vi "Dashboard Main.vi"() -> ()   [LabVIEW 2013]
uses:
  subStates.ctl
  <vilib>/event_ctls.llb/eventvkey.ctl
  dash dio.ctl
  misc dash data.ctl
  dashboard safety status data.ctl
  dash error type def.ctl
  <vilib>/Utility/config.llb/Write Key (String).vi
  <vilib>/Utility/config.llb/Write Key (I32).vi
  <vilib>/Utility/config.llb/NI_LVConfig.lvlib
panel:
  out "Image Message":string="Timeout in Camera Communications"
  in  "Dashboard Tab":T1(tab)
  out "no rate":bool
  out "arm encoder limit":bool
  out "hold":bool
  out "shoot?":bool
  out "Shifter":bool
  out "Vision State":bool
  in  "Camera Settings":T2={"Frame Rate"=30, "Compression"=30, "Size"=1} {"Frame Rate" scale=1.0..30.0; "Size" items=["640x480", "320x240", "160x120"]}
  out "Mode":T3(ring)=enum."Auto Disabled"
  out "Camera IP":string
  in  "DB Camera Config":bool
  out "fps":dbl format="%#.1g"
  out "Mbps":dbl format="%#.1g"
  out "Mbps 2":bool
  out "Distance From Target":dbl
  out "Hot Goal Present?":bool
  out "arm saftey":bool
  out "Directional Failure":bool
  out "timeout error":bool
  out "# of Timeouts":u32
  out "Robot IP\nAddress":string
  out "Solenoid Output":bool[](array[boolean])
  out "PWM":cluster{u8, u8}[](array[slide])=[{0, 157}, {0, 157}, {0, 157}, {0, 157}, {0, 157}, {0, 157}, {0, 157}, {0, 157}, {0, 157}, {0, 169}] scale=1.0..255.0
  out "GPIO Output Enable":bool[](array[boolean])
  out "GPIO State":bool[](array[boolean])
  out "Relay":cluster{"Forward":bool[], "Reverse":bool[]}
  out "8 -- Battery":sgl(graph)
  out "Analog Input":sgl[](array[slide]) scale=0.0..5.0
  out "Drive":T4
  out "Pickup/Passing \nArm":cluster{"Distance ":dbl, "Rate":dbl}
  out "Latch":T5
  out "Pickup Arm":T5
  out "Belts":T5
  out "Shooter":T5
  out "Drive":T5
  out "Belt Status":u16(ring) items=["Code Control", "Driver Control", "Manual Override"]
  out "Arm Status":u16(ring) items=["Code Control", "Driver Control", "Manual Override"]
  out "Belts":dbl
  out "CPU":dbl(slide) scale=0.0..100.0
  out "cRIO CPU Usage":dbl(knob) scale=0.0..100.0
  out "Code Iterations Per Second":cluster{dbl, dbl}(knob) scale=0.0..60.0
  out "Vision mSPI":u32
  out "Main mSPI":u32
  in  "Listbox":i32(listbox)
  out "Tree":string(tree)
  in  "Enable":bool
  # "ft"
  # "Encoders"
  # "States"
  # "Drive"
  # "Belts"
  # "Communications"
  # "Solenoid #1"
  # "1"
  # "8"
  # "Digital #1"
  # "1"
  # "10"
  # "1"
  # "14"
  # "1"
  # "8"
  # "Analog #1"
  # "1"
  # "7"
  # "Main IPS"
  # "Vision IPS"
  # "Grey - Vision\nBlack - Main"
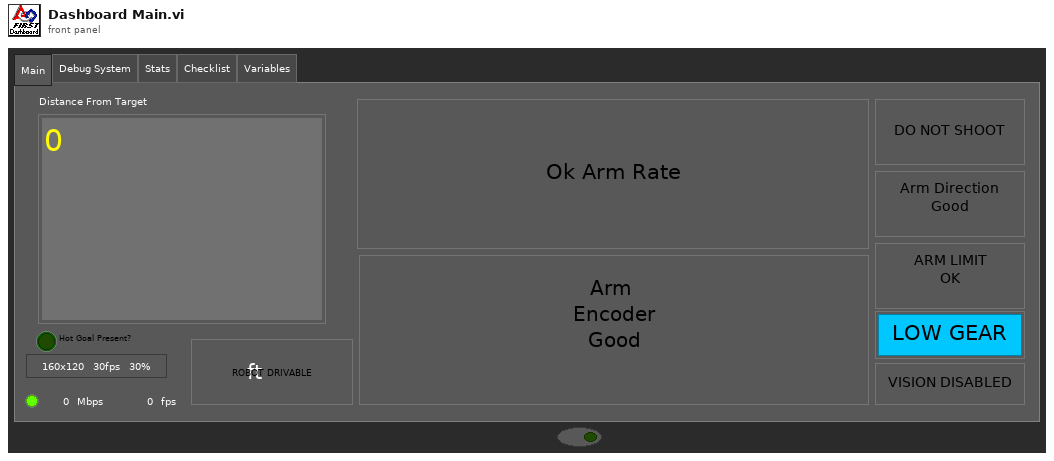
[diagram p1: front panel]
types:
  T1 = enum32{"Main", "Debug System", "Stats", "Checklist", "Variables"}
  T2 = cluster{"Frame Rate":i32, "Compression":i32, "Size":u16}
  T3 = enum8{"Tele-Op Disabled", "Tele-Op Enabled", "Auto Disabled", "Auto Enabled", "Test Disabled", "Test Enabled", ""}
  T4 = cluster{"Right Rate":dbl, "Left Rate":dbl, "Left Distance":dbl, "Right Distance":dbl}
  T5 = typedef "subStates.ctl" = enum16{"null", "wait", "driver control", "auto", "manual override", "hold position", "rotate", "pickup", "pass", "load", "goto shoot", "shoot", "end", "test"}
  T6 = typedef "Image Type" = u32
  T7 = typedef "IMAQ Image.ctl" = refnum<image>
  T8 = typedef "dash error type def.ctl" = cluster{"Timeout Data":cluster{"# of Timeouts":u32, "Time Out Error This Match":bool}, "Can Shoot Safely?":bool}
  T9 = typedef "misc dash data.ctl" = cluster{"Total (%)":dbl, "Vision mSPI":u32, "Main mSPI":u32, "Vision":cluster{"Hot Goal Present?":bool, "distance":dbl}, "Enabled?":bool, "Safety Data":T10}
  T10 = typedef "dashboard safety status data.ctl" = cluster{"At Distance Limit":bool, "Encoder Error":bool, "Excedded Rate Limit":bool, "Encoder Directional Issue":bool}
  T11 = typedef "dash dio.ctl" = cluster{"Relay Forward":u8, "Relay Reverse":u8, u32, u32, cluster{"[0]":u8, "[1]":u8, "[2]":u8, "[3]":u8, "[4]":u8, "[5]":u8, "[6]":u8, "[7]":u8, "[8]":u8, "[9]":u8}}[]
  T12 = cluster{"Digital Inputs":bool[], "Digital Outputs":bool[]}
  T13 = cluster{"Competition mode":bool, "Robot Link":bool, "Autonomous":bool, "Enabled":bool, "E-Stop":bool, "Simulated":bool, "TestMode":bool, "Docked Window":bool}
  T14 = cluster{"Relay Forward":u8, "Relay Reverse":u8, u32, u32, cluster{"[0]":u8, "[1]":u8, "[2]":u8, "[3]":u8, "[4]":u8, "[5]":u8, "[6]":u8, "[7]":u8, "[8]":u8, "[9]":u8}}
  T15 = cluster{"Hot Goal Present?":bool, "distance":dbl}
  T16 = cluster{"# of Timeouts":u32, "Time Out Error This Match":bool}
  T17 = cluster{"Numeric":dbl, "Numeric":dbl, "Numeric":dbl, "Numeric":dbl}
  T18 = typedef "NI_LVConfig.lvlib/Config Data RefNum.ctl" = refnum<k1>
  T19 = typedef "eventvkey.ctl" = enum16{"ASCII", "Enter", "Return", "Shift", "Ctrl", "Alt", "Cmd", "Opt", "Caps", "NumLock", "Clear", "Break", "Up", "Down", "Left", "Right", "Insert", "Delete", "Home", "End", "PageUp", "PageDown", "Escape", "Help", "Pause", "ScrollLock", "F1", "F2", "F3", "F4", "F5", "F6", "F7", "F8", "F9", "F10", "F11", "F12", "F13", "F14", "F15", "F16", "F17", "F18", "F19", "F20", "F21", "F22", "F23", "F24", "Play", "VolumeUp", "VolumeDown", "Mute", "Two Byte Char"}
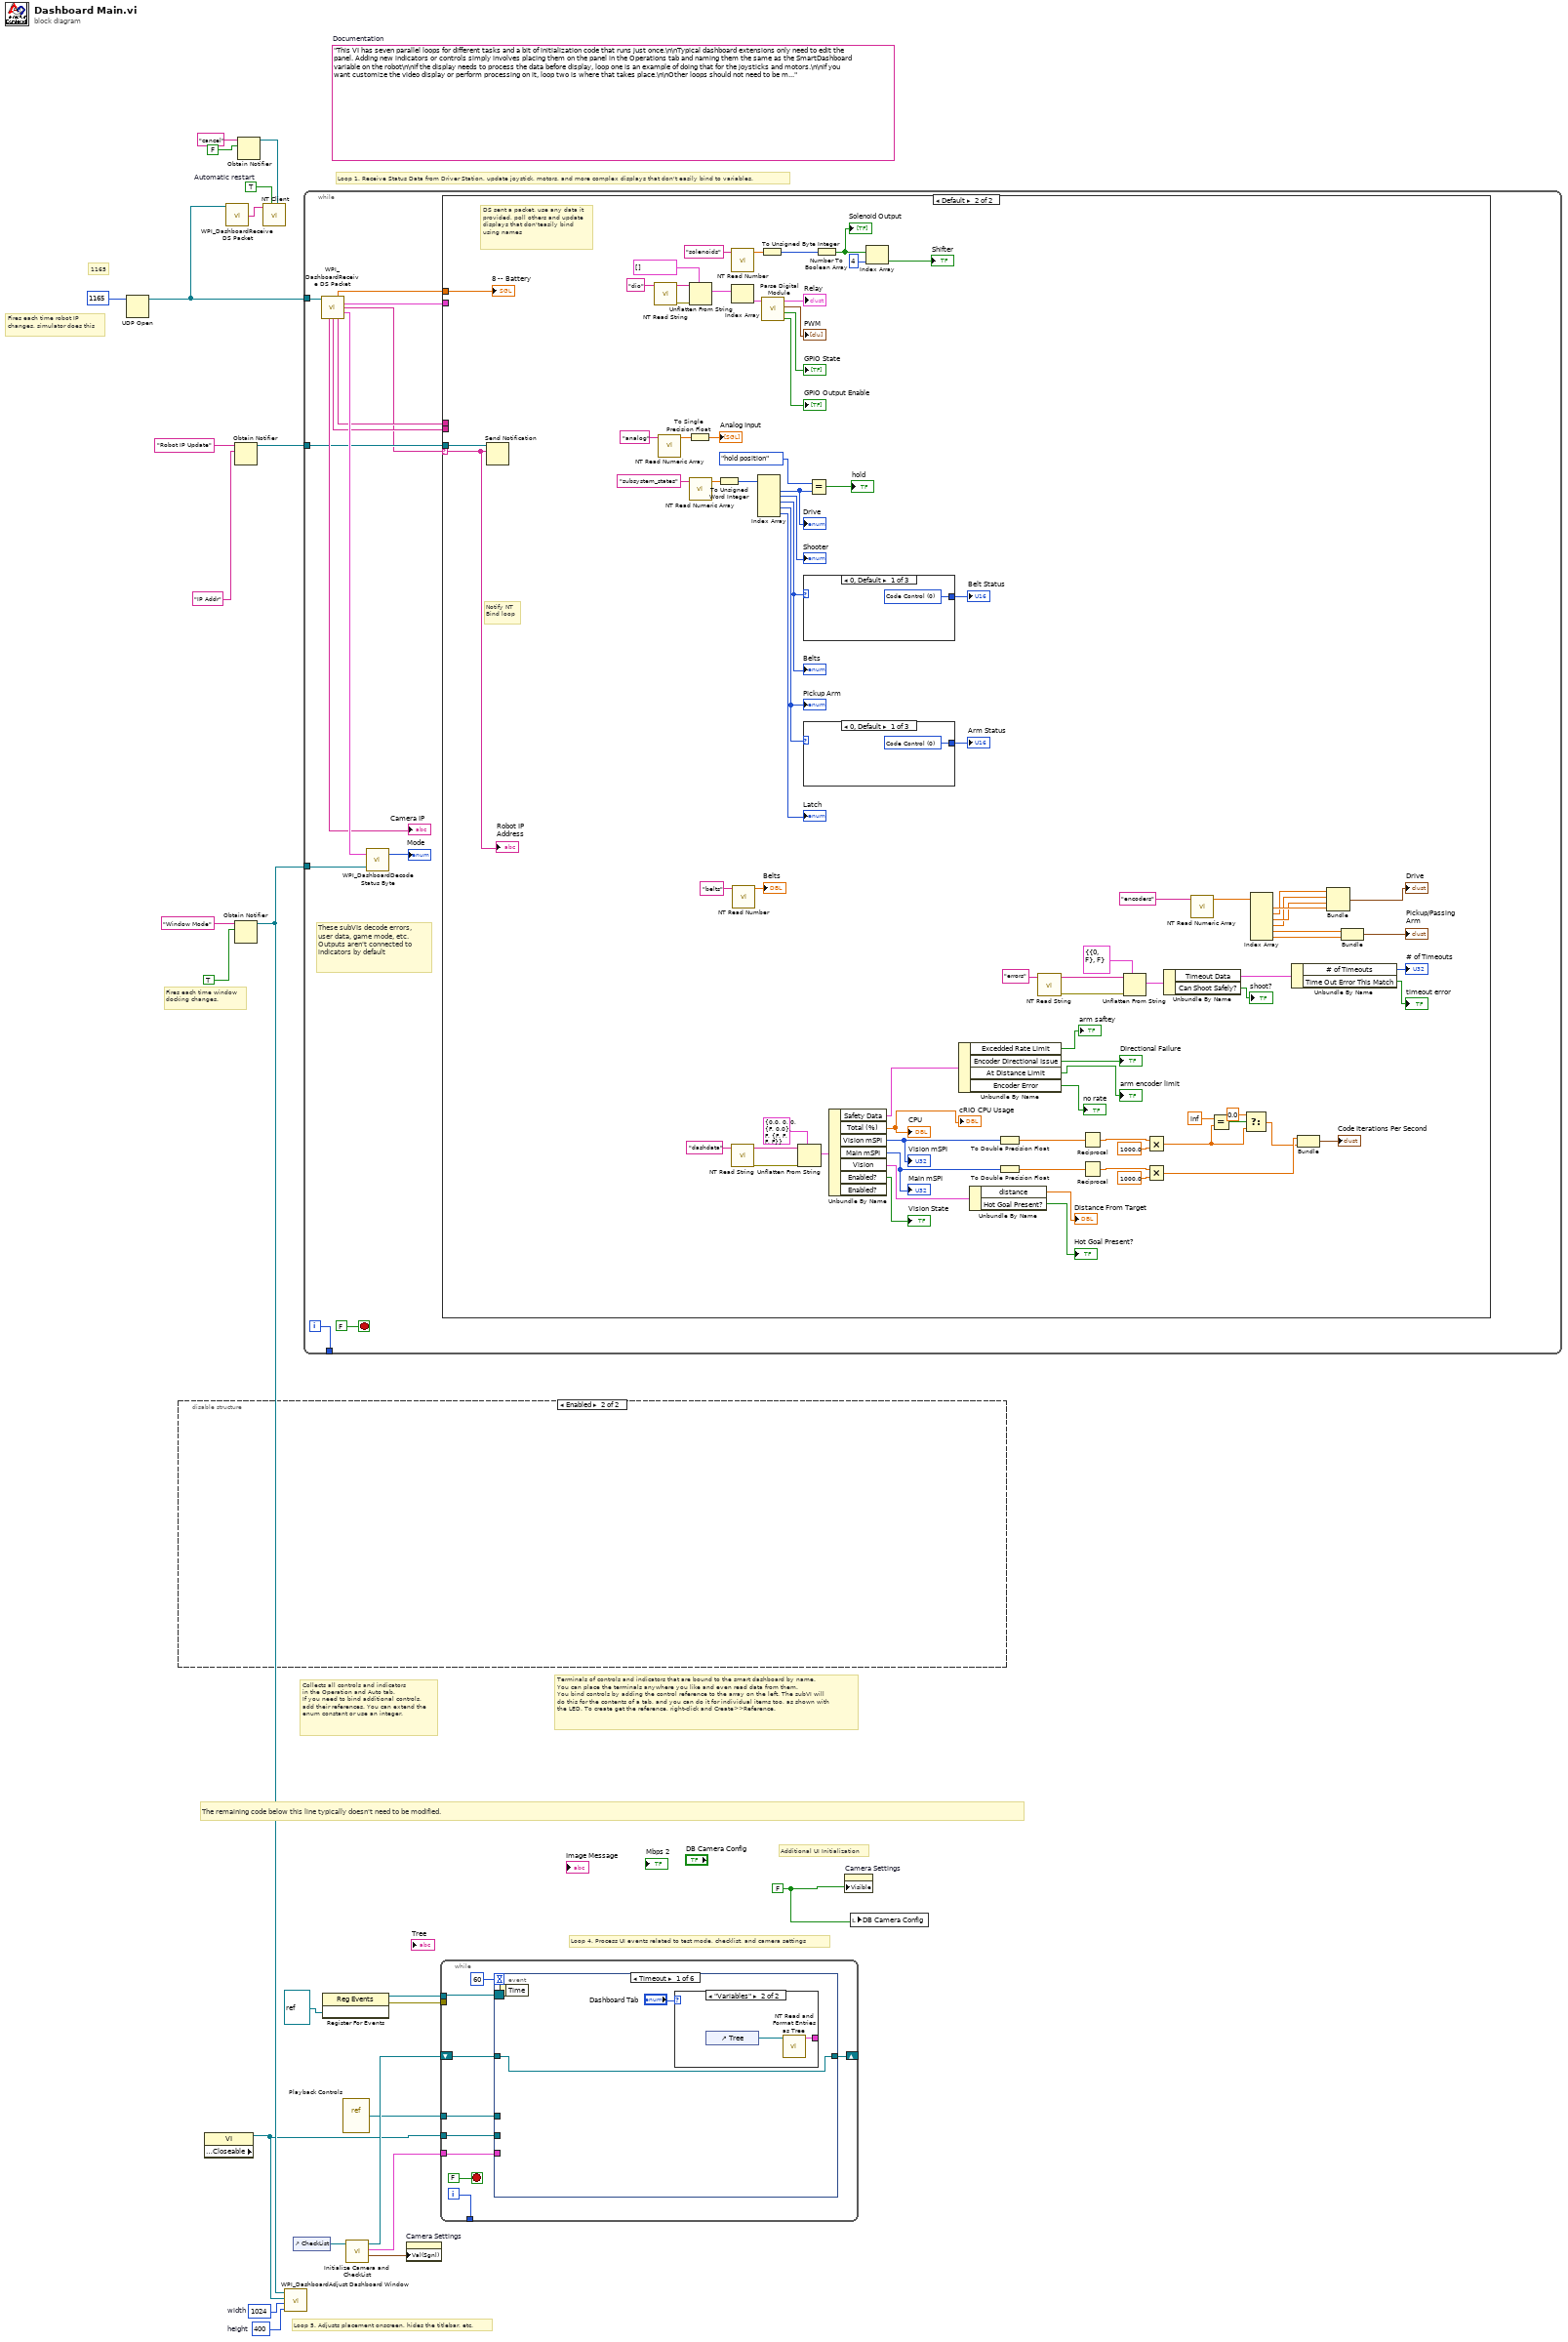
[diagram p0: block diagram]
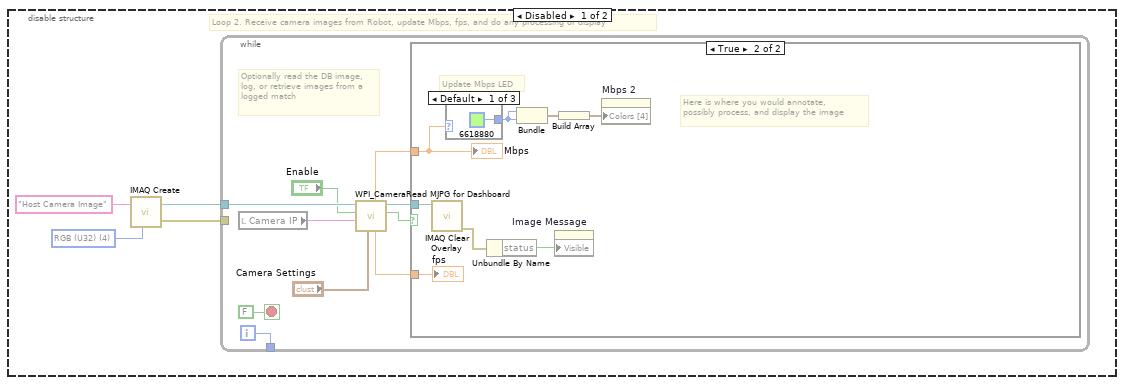
[diagram p2: hidden frame]
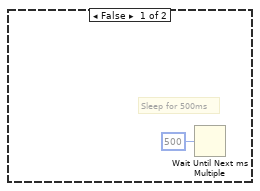
[diagram p3: hidden frame]
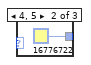
[diagram p4: hidden frame]
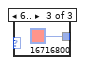
[diagram p5: hidden frame]
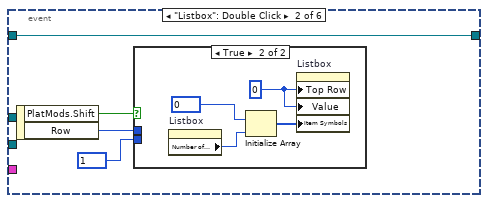
[diagram p7: hidden frame]
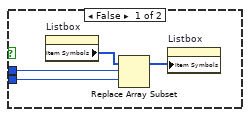
[diagram p8: hidden frame]
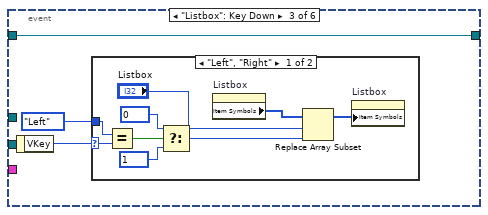
[diagram p9: hidden frame]
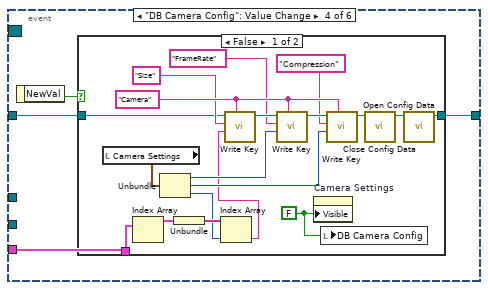
[diagram p11: hidden frame]
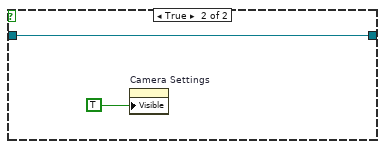
[diagram p12: hidden frame]
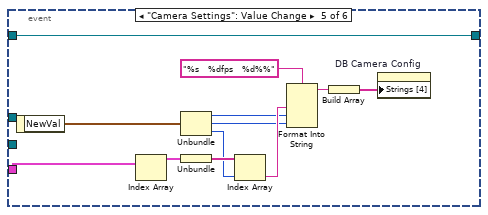
[diagram p13: hidden frame]
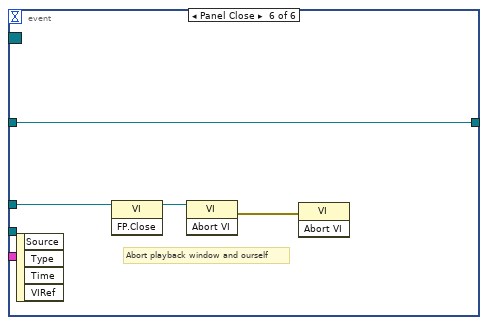
[diagram p14: hidden frame]
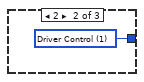
[diagram p16: hidden frame]
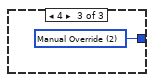
[diagram p17: hidden frame]
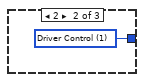
[diagram p18: hidden frame]
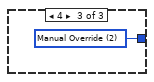
[diagram p19: hidden frame]
diagram:
  w6 = TRUE  # Automatic restart
  w9 = 400  # height
  w10 = 1024  # width
  w19 = FALSE ("Visible")
  (unwired) "This VI has seven parallel loops for different tasks and a bit of initialization code that runs just once.\n\nTypical dashboard extensions only need to edit the panel. Adding new indicators or controls simply involves placing them on the panel in the Operations tab and naming them the same as the SmartDashboard variable on the robot\n\nIf the display needs to process the data before display, loop one is an example of doing that for the joysticks and motors.\n\nIf you want customize the video display or perform processing on it, loop two is where that takes place.\n\nOther loops should not need to be modified. They are pretty standard, and document the task they perform."  # Documentation
  # "1165"
  # "Loop 4. Process UI events related to test mode, checklist, and camera settings"
  # "Loop 5. Adjusts placement onscreen, hides the titlebar, etc."
  # "Additional UI Initialization"
  # "Fires each time robot IP\nchanges, simulator does this"
  # "Fires each time window\ndocking changes."
  # "Collects all controls and indicators\nin the Operation and Auto tab.\nIf you need to bind additional controls,\nadd their references. You can extend the\nenum constant or use an integer."
  # "The remaining code below this line typically doesn't need to be modified."
  # "Terminals of controls and indicators that are bound to the smart dashboard by name.\nYou can place the terminals anywhere you like and even read data from them.\nYou bind controls by adding the control reference to the array on the left. The subVI will\ndo this for the contents of a tab, and you can do it for individual items too, as shown with\nthe LED. To create get the reference, right-click and Create>>Reference."
  # "Loop 1. Receive Status Data from Driver Station, update joystick, motors, and more complex displays that don't easily bind to variables."
  n1 = UDP Open(11:u16 1165 ("port")) -> (port=w1:refnum<k16>)  [unwired: 2 in, 4 out]
  n2 = disable-structure shown="Enabled" {
    frame Disabled {
      w29 = T6 4 items=["Grayscale (U8)", "Grayscale (I16)", "Grayscale (SGL)", "Complex (CSG)", "RGB (U32)", "HSL (U32)", "RGB (U64)"] ("Image Type")
      # "Loop 2. Receive camera images from Robot, update Mbps, fps, and do any processing or display"
      n3 = call "IMAQ Create"("Image Name"="Host Camera Image", "Image Type"=w29) -> ("New Image"=w27:T7, "error out"=w26:errorcluster)  [unwired: 2 in, 1 out]
      n4 = while {
        tunnel: w27 -> [w37]
        tunnel: w26 -> [_]
        tunnel: [w38] -> _
        i -> [w38]
        stop <- FALSE stop-if-true
        # "Optionally read the DB image,\nlog, or retrieve images from a\nlogged match"
        n5 = local read "Camera IP"() -> (w30:string)
        n6 = call <vilib>:"WPI_CameraRead MJPG for Dashboard.vi"("Camera Settings"="Camera Settings", "Camera IP"=w30, "Enable"="Enable", "Refnum in"=w37) -> ("Active"=w34:bool, "Refnum out"=w36:T7, "FPS"=w33:dbl, "Bandwidth (Mbps)"=w32:dbl)  [unwired: 4 in]
        n7 = case shown="True" w34 {
          tunnel: w36 -> [_ w44]
          tunnel: w32 -> [_ w43]
          tunnel: w33 -> [_ w41]
          frame False {
            # "Sleep for 500ms"
            n8 = Wait Until Next ms Multiple(millisecond multiple=u32 500) -> ()  [unwired: 1 out]
          }
          frame True {
            # "Here is where you would annotate,\npossibly process, and display the image"
            # "Update Mbps LED"
            n9 = call "IMAQ Clear Overlay"("Image"=w44) -> ("error out"=w48:errorcluster, "Image Out"=w42:T7)  [unwired: 2 in, 7 out]
            n10 = case shown="Default" w43 {
              tunnel: [u32 6618880 ("Color Box") u32 16776722 ("Color Box") u32 16716800 ("Color Box")] -> w45
              frame Default {
              }
              frame 4, 5 {
              }
              frame 6.. {
              }
            }
            n11 = Unbundle By Name(w48) -> ("status"=w49:bool)
            n12 = Bundle("Color Box"=w45, "Color Box"=w45) -> (w47:cluster{"Color Box":u32, "Color Box":u32})  [unwired: 1 out]
            n13 = property on="Image Message" class="Str"("Visible"=w49) -> ()  [unwired: 2 in, 2 out]
            n14 = Build Array(w47) -> (w46:cluster{"Color Box":u32, "Color Box":u32}[])
            n15 = property on="Mbps 2" class="Bool (strict)"("Colors [4]"=w46) -> ()  [unwired: 2 in, 2 out]
            "Mbps" <- w43
            "fps" <- w41
          }
        }
      }
    }
    frame Enabled {
    }
  }
  n16 = property class="VI" props=["Front Panel.Closeable"]() -> (reference out=w7:refnum<vi>)  [unwired: 2 in, 2 out]
  n17 = call <vilib>:"WPI_DashboardReceive DS Packet.vi"("Recv Socket"=w1) -> ("Robot IP Address"=w2:string)  [unwired: 1 in, 13 out]
  n18 = Obtain Notifier(name (unnamed)="Robot IP Update", notification data type="IP Addr" ("name (unnamed)")) -> (notifier out=w22:refnum<notifier>)  [unwired: 2 in, 2 out]
  n19 = Obtain Notifier(name (unnamed)="Window Mode", notification data type=TRUE) -> (notifier out=w18:refnum<notifier>)  [unwired: 2 in, 2 out]
  n20 = Obtain Notifier(name (unnamed)="cancel", notification data type=FALSE) -> (notifier out=w3:refnum<notifier>)  [unwired: 2 in, 2 out]
  n21 = call <vilib>:"NT Client.vi"("Cancel Ref"=w3, "Automatic restart"=w6, "Server IP Address"=w2) -> ()  [unwired: 9 in]
  n22 = call <vilib>:"WPI_DashboardAdjust Dashboard Window.vi"("height"=w9, "width"=w10, "reference in"=w7, "Notifier in"=w18) -> ()  [unwired: 8 in]
  n23 = control-ref of="CheckList"() -> (w8:refnum<vi>)
  n24 = while {
    tunnel: w1 -> [w63]
    tunnel: w22 -> [w58]
    tunnel: w18 -> [w62]
    tunnel: [w59] -> _
    i -> [w59]
    stop <- FALSE stop-if-true
    # "These subVIs decode errors, user data, game mode, etc.\nOutputs aren't connected to indicators by default"
    n25 = call <vilib>:"WPI_DashboardReceive DS Packet.vi"("Recv Socket"=w63) -> ("Battery"=w54:sgl, "Driver Station"=w55:T12, "Robot IP Address"=w53:string, "Status"=w64:T13, "Camera IP Address"=→"Camera IP":string, "Low Priority User Data"=w57:string, "High Priority User Data"=w56:string)  [unwired: 1 in, 7 out]
    n26 = call <vilib>:"WPI_DashboardDecode Status Byte.vi"("Window Mode Notifier"=w62, "Status"=w64) -> ("Mode"=→"Mode":T3)  [unwired: 1 out]
    n27 = case shown="Default" w53 {
      selector: w53 -> [_ w74]
      tunnel: w58 -> [_ w150]
      tunnel: w57 -> [_ _]
      tunnel: w56 -> [_ _]
      tunnel: w55 -> [_ _]
      tunnel: w54 -> [_ w125]
      frame "0.0.0.0" {
        # "DS not sending packets, or no robot exists yet.\nDon't poll the variables"
      }
      frame Default {
        # "Notify NT\nBind loop"
        # "DS sent a packet. use any data it\nprovided, poll others and update\ndisplays that don'teasily bind\nusing names"
        n28 = Send Notification(notification=w74, notifier=w150) -> ()  [unwired: 1 in, 2 out]
        n29 = call <vilib>:"NT Read String.vi"("Name"="dio") -> ("error out"=w114:errorcluster, "String"=w116:string)  [unwired: 9 in]
        n30 = call <vilib>:"NT Read Numeric Array.vi"("Name"="analog") -> ("Numeric Array"=w127:dbl[])  [unwired: 9 in, 1 out]
        n31 = To Single Precision Float(number=w127) -> (single precision float=→"Analog Input":sgl[])
        n32 = call <vilib>:"NT Read Numeric Array.vi"("Name"="subsystem_states") -> ("Numeric Array"=w123:dbl[])  [unwired: 9 in, 1 out]
        n33 = Unflatten From String(type=T11 [] ("array"), binary string=w116, error in (no error)=w114) -> (value=w113:T11)  [unwired: 2 in, 2 out]
        n34 = To Unsigned Word Integer(number=w123) -> (unsigned 16bit integer=w122:u16[])
        n35 = call <vilib>:"NT Read Number.vi"("Name"="solenoids") -> ("Numeric"=w110:dbl)  [unwired: 9 in, 1 out]
        n36 = Index Array(array=w113) -> (element=w112:T14)  [unwired: 1 in]
        n37 = call <vilib>:"NT Read String.vi"("Name"="dashdata") -> ("error out"=w96:errorcluster, "String"=w95:string)  [unwired: 9 in]
        n38 = call <vilib>:"NT Read Number.vi"("Name"="belts") -> ("Numeric"=→"Belts":dbl)  [unwired: 9 in, 1 out]
        n39 = Index Array(array=w122) -> (element #1=w107:u16, element #2=→"Shooter":u16, element #3=w119:u16, element #4=w120:u16, element #5=→"Latch":u16)  [unwired: 5 in]
        "Drive" <- w107
        "Belts" <- w119
        "Pickup Arm" <- w120
        n40 = To Unsigned Byte Integer(number=w110) -> (unsigned 8bit integer=w109:u8)
        n41 = call "Parse Digital Module.vi"("DigitalModule"=w112) -> ("GPIO Output Enable"=→"GPIO Output Enable":bool[], "GPIO State"=→"GPIO State":bool[], "PWM"=→"PWM":cluster{u8, u8}[], "Relay"=→"Relay":cluster{"Forward":bool[], "Reverse":bool[]})  [unwired: 7 in]
        n42 = Unflatten From String(type=T9 {"Total (%)"=0.0, "Vision mSPI"=0, "Main mSPI"=0, "Vision"={"Hot Goal Present?"=FALSE, "distance"=0.0}, "Enabled?"=FALSE, "Safety Data"={"At Distance Limit"=FALSE, "Encoder Error"=FALSE, "Excedded Rate Limit"=FALSE, "Encoder Directional Issue"=FALSE}} ("Misc Dash Data"), binary string=w95, error in (no error)=w96) -> (value=w93:T9)  [unwired: 2 in, 2 out]
        n43 = case shown="0, Default" w119 {
          tunnel: [w151 w152 w153] -> w132
          frame 0, Default {
            w151 = u16 0 items=["Code Control", "Driver Control", "Manual Override"] ("Arm Status")
          }
          frame 2 {
            w152 = u16 1 items=["Code Control", "Driver Control", "Manual Override"] ("Arm Status")
          }
          frame 4 {
            w153 = u16 2 items=["Code Control", "Driver Control", "Manual Override"] ("Arm Status")
          }
        }
        "Belt Status" <- w132
        n44 = case shown="0, Default" w120 {
          tunnel: [w154 w155 w156] -> w131
          frame 0, Default {
            w154 = u16 0 items=["Code Control", "Driver Control", "Manual Override"] ("Arm Status")
          }
          frame 2 {
            w155 = u16 1 items=["Code Control", "Driver Control", "Manual Override"] ("Arm Status")
          }
          frame 4 {
            w156 = u16 2 items=["Code Control", "Driver Control", "Manual Override"] ("Arm Status")
          }
        }
        "Arm Status" <- w131
        n45 = Equal?(x=subStates."hold position" ("Drive"), y=w107) -> (x = y?=→"hold":bool)
        n46 = Number To Boolean Array(number=w109) -> (Boolean array=w108:bool[])
        "Solenoid Output" <- w108
        n47 = Unbundle By Name(w93) -> ("Safety Data"=w89:T10, "Total (%)"=→"cRIO CPU Usage" →"CPU":dbl, "Vision mSPI"=w87:u32, "Main mSPI"=w88:u32, "Vision"=w92:T15, "Enabled?"=→"Vision State":bool)  [unwired: 1 out]
        "Vision mSPI" <- w87
        "Main mSPI" <- w88
        n48 = Index Array(array=w108, index=4) -> (element=→"Shifter":bool)
        n49 = Unbundle By Name(w89) -> ("Excedded Rate Limit"=→"arm saftey":bool, "Encoder Directional Issue"=→"Directional Failure":bool, "At Distance Limit"=→"arm encoder limit":bool, "Encoder Error"=→"no rate":bool)
        n50 = Unbundle By Name(w92) -> ("distance"=→"Distance From Target":dbl, "Hot Goal Present?"=→"Hot Goal Present?":bool)
        n51 = To Double Precision Float(number=w87) -> (double precision float=w136:dbl)
        n52 = To Double Precision Float(number=w88) -> (double precision float=w141:dbl)
        n53 = call <vilib>:"NT Read String.vi"("Name"="errors") -> ("error out"=w102:errorcluster, "String"=w101:string)  [unwired: 9 in]
        n54 = Reciprocal(x=w136) -> (1/x=w137:dbl)
        n55 = Reciprocal(x=w141) -> (1/x=w140:dbl)
        n56 = Unflatten From String(type=T8 {"Timeout Data"={"# of Timeouts"=0, "Time Out Error This Match"=FALSE}, "Can Shoot Safely?"=FALSE} ("Errors"), binary string=w101, error in (no error)=w102) -> (value=w99:T8)  [unwired: 2 in, 2 out]
        n57 = Multiply(x=w137, y=1000.0) -> (x*y=w71:dbl)
        n58 = Multiply(x=w140, y=1000.0) -> (x*y=w135:dbl)
        n59 = Unbundle By Name(w99) -> ("Timeout Data"=w97:T16, "Can Shoot Safely?"=→"shoot?":bool)
        n60 = call <vilib>:"NT Read Numeric Array.vi"("Name"="encoders") -> ("Numeric Array"=w86:dbl[])  [unwired: 9 in, 1 out]
        n61 = Equal?(x=inf, y=w71) -> (x = y?=w72:bool)
        n62 = Select(t=0.0, s=w72, f=w71) -> (s? t:f=w70:dbl)
        n63 = Index Array(array=w86) -> (element #1=w85:dbl, element #2=w84:dbl, element #3=w83:dbl, element #4=w82:dbl, element #5=w81:dbl, element #6=w80:dbl)  [unwired: 6 in]
        n64 = Unbundle By Name(w97) -> ("# of Timeouts"=→"# of Timeouts":u32, "Time Out Error This Match"=→"timeout error":bool)
        n65 = Bundle(w135, "t"=w70) -> (→"Code Iterations Per Second":cluster{dbl, "t":dbl})  [unwired: 1 in]
        n66 = Bundle("Numeric"=w84, "Numeric"=w82, "Numeric"=w83, "Numeric"=w85) -> (→"Drive":T17)  [unwired: 1 in]
        n67 = Bundle("Numeric"=w81, "Numeric"=w80) -> (→"Pickup/Passing \nArm":cluster{"Numeric":dbl, "Numeric":dbl})  [unwired: 1 in]
        "8 -- Battery" <- w125
        "Robot IP\nAddress" <- w74
      }
    }
  }
  n68 = register-events(refnum<vi> refnum) -> (reference out=w13:refnum<event-registration>, error out=w12:errorcluster)  [unwired: 2 in]
  n69 = vi-ref "Playback Controls.vi"() -> (w14:refnum<vi>)
  n70 = call "Initialize Camera and CheckList.vi"("ListBox in"=w8) -> ("Cluster"=w16:cluster{"value":i32, "value":i32, "index":i32}, "Array"=w17:cluster{string[]}[], "File Refnum"=w15:T18)  [unwired: 8 in]
  n71 = property on="Camera Settings" class="Clust (strict)"("Val(Sgnl)"=w16) -> ()  [unwired: 2 in, 2 out]
  n72 = while {
    tunnel: w17 -> [w163]
    shift-right: [w162] -> _
    shift-left: w15 -> [w161]
    tunnel: [w160] -> _
    tunnel: w14 -> [w159]
    tunnel: w13 -> [w158]
    tunnel: w12 -> [_]
    tunnel: w7 -> [w157]
    i -> [w160]
    stop <- FALSE stop-if-true
    n73 = event shown="[0] Timeout" {
      selector: w158 -> [_ _ _ _ _ _]
      dyn-events: _ -> [_ _ _ _ _ _]
      timeout: u32 60 ("milliseconds to wait") -> [_ _ _ _ _ _]
      tunnel: w163 -> [_ _ _ w196 w226 _]
      tunnel: [w166 w170 w182 w195 w219 w231] -> w162
      tunnel: w161 -> [w166 w170 w182 w194 w219 w231]
      tunnel: w159 -> [_ _ _ _ _ w234]
      tunnel: w157 -> [_ _ _ _ _ _]
      event Timeout {
        n74 = event-data() -> ()  [unwired: 1 in, 1 out]
        n75 = case shown="\"Variables\"" "Dashboard Tab" {
          tunnel: [_ w169] -> _
          frame "Debug System", Default {
          }
          frame "Variables" {
            n76 = control-ref of="Tree"() -> (w168:refnum<vi>)
            n77 = call <vilib>:"NT Read and Format Entries as Tree.vi"("Tree Refnum"=w168) -> ("Formatted Strings"=w169:cluster{"Name":string, "Value":string}[])  [unwired: 9 in, 1 out]
          }
        }
      }
      event "Listbox": Double Click {
        n78 = event-data() -> ("PlatMods.Shift"=w171:bool, "Row"=w173:i32)  [unwired: 1 in]
        n79 = case shown="True" w171 {
          tunnel: w173 -> [w177 _]
          tunnel: 1 -> [w176 _]
          frame False {
            n80 = property on="Listbox" class="LstBox (strict)"() -> ("Item Symbols"=w175:i32[])  [unwired: 2 in, 2 out]
            n81 = Replace Array Subset(array=w175, new element=w176, index=w177) -> (w174:i32[])
            n82 = property on="Listbox" class="LstBox (strict)"("Item Symbols"=w174) -> ()  [unwired: 2 in, 2 out]
          }
          frame True {
            w178 = 0 ("Top Row")
            n83 = property on="Listbox" class="LstBox (strict)"() -> ("Number of Rows"=w180:u32)  [unwired: 2 in, 2 out]
            n84 = Initialize Array(0, w180) -> (w179:i32[])
            n85 = property on="Listbox" class="LstBox (strict)"("Top Row"=w178, "Value"=w178, "Item Symbols"=w179) -> ()  [unwired: 2 in, 2 out]
          }
        }
      }
      event "Listbox": Key Down {
        n86 = event-data() -> ("VKey"=w184:T19)  [unwired: 1 in]
        n87 = case shown="\"Left\", \"Right\"" w184 {
          selector: w184 -> [w189 _]
          tunnel: eventvkey."Left" ("VKey") -> [w187 _]
          frame "Left", "Right" {
            n88 = Equal?(x=w187, y=w189) -> (x = y?=w188:bool)
            n89 = Select(t=0, s=w188, f=1) -> (s? t:f=w190:i32)
            n90 = property on="Listbox" class="LstBox (strict)"() -> ("Item Symbols"=w193:i32[])  [unwired: 2 in, 2 out]
            n91 = Replace Array Subset(array=w193, new element=w190, index="Listbox") -> (w192:i32[])
            n92 = property on="Listbox" class="LstBox (strict)"("Item Symbols"=w192) -> ()  [unwired: 2 in, 2 out]
          }
          frame Default {
          }
        }
      }
      event "DB Camera Config": Value Change {
        n93 = event-data() -> ("NewVal"=w197:bool)  [unwired: 1 in]
        n94 = case shown="False" w197 {
          tunnel: w196 -> [w206 _]
          tunnel: [w199 w217] -> w195
          tunnel: w194 -> [w198 w217]
          frame False {
            w213 = "Camera"
            w216 = FALSE ("Visible")
            n95 = local read "Camera Settings"() -> (w205:T2)
            n96 = Index Array(array=w206) -> (element=w209:cluster{string[]})  [unwired: 1 in]
            n97 = Unbundle(w205) -> ("Frame Rate"=w204:i32, "Compression"=w203:i32, "Size"=w207:u16)
            n98 = Unbundle(w209) -> (w208:string[])
            n99 = Index Array(array=w208, index=w207) -> (element=w202:string)
            n100 = call-poly <vilib>:"Write Key.vi"("section"=w213, "value"=w202, "key"="Size", "refnum"=w198) -> ("refnum out"=w215:T18)  [unwired: 2 in, 5 out]
            n101 = call-poly <vilib>:"Write Key.vi"("section"=w213, "value"=w204, "key"="FrameRate", "refnum"=w215) -> ("refnum out"=w214:T18)  [unwired: 1 in, 6 out]
            n102 = property on="Camera Settings" class="Clust (strict)"("Visible"=w216) -> ()  [unwired: 2 in, 2 out]
            n103 = local write "DB Camera Config"(w216) -> ()
            n104 = call-poly <vilib>:"Write Key.vi"("section"=w213, "value"=w203, "key"="Compression", "refnum"=w214) -> ("refnum out"=w200:T18)  [unwired: 1 in, 6 out]
            n105 = call <vilib>:"Close Config Data.vi"("refnum"=w200) -> ("file path"=w201:path)  [unwired: 2 in, 8 out]
            n106 = call <vilib>:"Open Config Data.vi"("configuration file path"=w201) -> ("refnum"=w199:T18)  [unwired: 8 in, 2 out]
          }
          frame True {
            n107 = property on="Camera Settings" class="Clust (strict)"("Visible"=TRUE) -> ()  [unwired: 2 in, 2 out]
          }
        }
      }
      event "Camera Settings": Value Change {
        n108 = event-data() -> ("NewVal"=w230:T2)  [unwired: 1 in]
        n109 = Index Array(array=w226) -> (element=w225:cluster{string[]})  [unwired: 1 in]
        n110 = Unbundle(w230) -> ("Frame Rate"=w221:i32, "Compression"=w220:i32, "Size"=w223:u16)
        n111 = Unbundle(w225) -> (w224:string[])
        n112 = Index Array(array=w224, index=w223) -> (element=w222:string)
        n113 = Format Into String(format string="%s   %dfps   %d%%", w222, w221, w220) -> (resulting string=w227:string)  [unwired: 2 in, 1 out]
        n114 = Build Array(w227) -> (w228:string[])
        n115 = property on="DB Camera Config" class="Bool (strict)"("Strings [4]"=w228) -> ()  [unwired: 2 in, 2 out]
      }
      event Panel Close {
        # "Abort playback window and ourself"
        n116 = event-data() -> ()  [unwired: 1 in, 4 out]
        n117 = invoke class="VI" method="FP.Close"(reference=w234) -> (reference out=w233:refnum<vi>)  [unwired: 2 in, 2 out]
        n118 = invoke class="VI" method="Abort VI"(reference=w233) -> (error out=w232:errorcluster)  [unwired: 2 in, 2 out]
        n119 = invoke class="VI" method="Abort VI"(error in=w232) -> ()  [unwired: 2 in, 3 out]
      }
    }
  }
  n120 = property on="Camera Settings" class="Clust (strict)"("Visible"=w19) -> ()  [unwired: 2 in, 2 out]
  n121 = local write "DB Camera Config"(w19) -> ()
